vi "字符串01至布尔转换.vi"(11 "字符串":string) -> (3 "布尔值":bool)   [LabVIEW 2013]
uses:
  <vilib>/Utility/error.llb/whitespace.ctl
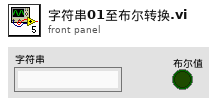
[diagram p1: front panel]
types:
  T1 = typedef "whitespace.ctl" = u16
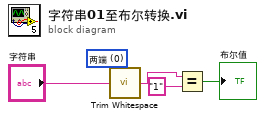
[diagram p0: block diagram]
diagram:
  w4 = T1 0 items=["两端", "字符串首端", "字符串末端"] ("location (both)")
  n1 = call <vilib>:"Trim Whitespace.vi"("string"="字符串", "location (both)"=w4) -> ("trimmed string"=w3:string)
  n2 = Equal?(x=w3, y="1") -> (x = y?=→"布尔值":bool)
